vi "GetInstVisaHandle.vi"(8 "error in (no error)":errorcluster, 11 "PwrMtr_RSNRPZ in":refnum<class "PwrMtr_RSNRPZ.lvclass">) -> (0 "error out":errorcluster, 2 "VISA resource name out":refnum<visa-resource-name>, 3 "PwrMtr_RSNRPZ out":refnum<class "PwrMtr_RSNRPZ.lvclass">)   [LabVIEW 2014, in "PwrMtr_RSNRPZ.lvclass"]
uses:
  PwrMtr_RSNRPZ.lvclass
  PwrMtr_RSNRPZ.lvclass/PwrMtr_RSNRPZ.ctl
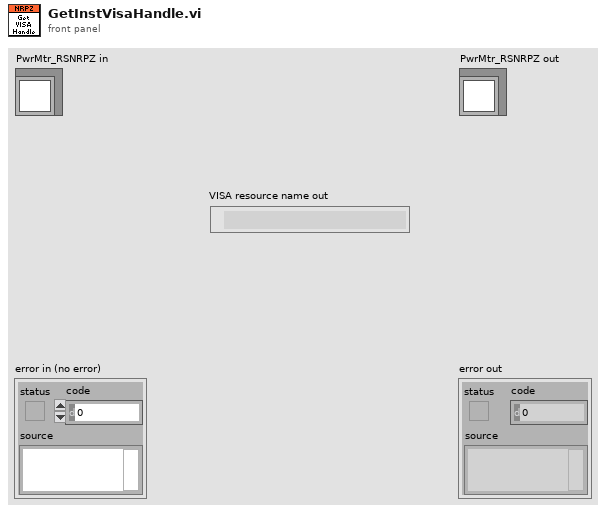
[diagram p1: front panel]
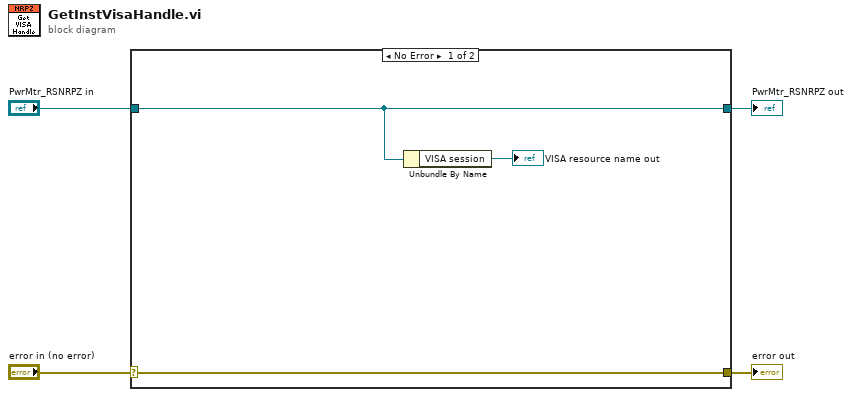
[diagram p0: block diagram]
diagram:
  n1 = case shown="No Error" "error in (no error)" {
    selector: "error in (no error)" -> [w7 w9]
    tunnel: [w7 w9] -> w3
    tunnel: [w6 w8] -> w1
    tunnel: "PwrMtr_RSNRPZ in" -> [w6 w8]
    frame No Error {
      n2 = Unbundle By Name(w6) -> ("VISA session"=→"VISA resource name out":refnum<visa-resource-name>)
    }
    frame Error {
    }
  }
  "error out" <- w3
  "PwrMtr_RSNRPZ out" <- w1
